vi "Task Manager.vi"(8 "error in (no error)":errorcluster, 11 "Task":string) -> (0 "error out":errorcluster, 3 "Task Properties":T1)   [LabVIEW 2018, in "Main.lvlib"]
uses:
  Main.lvlib
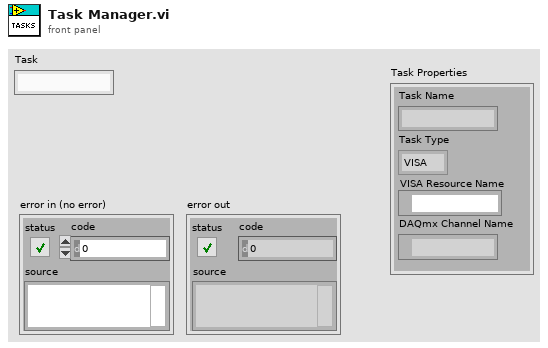
[diagram p1: front panel]
types:
  T1 = cluster{"Task Name":string, "Task Type":enum16{"VISA", "DAQmx"}, "VISA Resource Name":refnum<visa-resource-name>, "DAQmx Channel Name":tag}
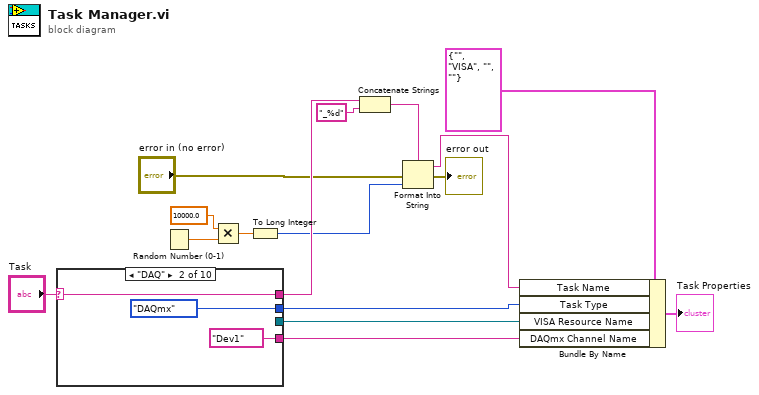
[diagram p0: block diagram]
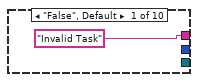
[diagram p2: hidden frame]
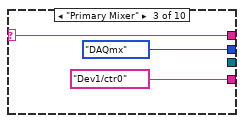
[diagram p3: hidden frame]
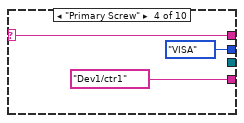
[diagram p4: hidden frame]
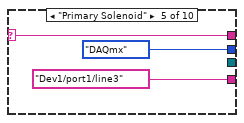
[diagram p5: hidden frame]
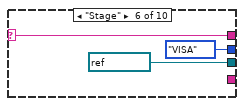
[diagram p6: hidden frame]
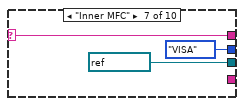
[diagram p7: hidden frame]
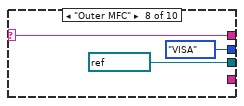
[diagram p8: hidden frame]
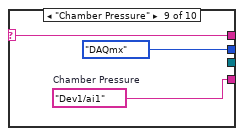
[diagram p9: hidden frame]
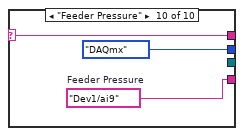
[diagram p10: hidden frame]
diagram:
  n1 = case shown="\"DAQ\"" "Task" {
    selector: "Task" -> [_ w20 w23 w26 w29 w32 w35 w38 w41 w44]
    tunnel: ["Invalid Task" w20 w23 w26 w29 w32 w35 w38 w41 w44] -> w15
    tunnel: [_ _ _ _ _ refnum<visa-resource-name> "COM8" ("VISA resource name") refnum<visa-resource-name> "COM2" ("VISA resource name") refnum<visa-resource-name> "COM1" ("VISA resource name") _ _] -> w4
    tunnel: [_ enum16{"VISA", "DAQmx"}."DAQmx" ("Task Type") enum16{"VISA", "DAQmx"}."DAQmx" ("Task Type") enum16{"VISA", "DAQmx"}."VISA" ("Task Type") enum16{"VISA", "DAQmx"}."DAQmx" ("Task Type") enum16{"VISA", "DAQmx"}."VISA" ("Task Type") enum16{"VISA", "DAQmx"}."VISA" ("Task Type") enum16{"VISA", "DAQmx"}."VISA" ("Task Type") enum16{"VISA", "DAQmx"}."DAQmx" ("Task Type") enum16{"VISA", "DAQmx"}."DAQmx" ("Task Type")] -> w3
    tunnel: [_ tag "Dev1" ("Counter(s)") tag "Dev1/ctr0" ("Counter(s)") tag "Dev1/ctr1" ("Counter(s)") tag "Dev1/port1/line3" ("lines") _ _ _ w40 w43] -> w2
    frame "False", Default {
    }
    frame "DAQ" {
    }
    frame "Primary Mixer" {
    }
    frame "Primary Screw" {
    }
    frame "Primary Solenoid" {
    }
    frame "Stage" {
    }
    frame "Inner MFC" {
    }
    frame "Outer MFC" {
    }
    frame "Chamber Pressure" {
      w40 = tag "Dev1/ai1"  # Chamber Pressure
    }
    frame "Feeder Pressure" {
      w43 = tag "Dev1/ai9"  # Feeder Pressure
    }
  }
  n2 = Random Number (0-1)() -> (number: 0 to 1=w14:dbl)
  n3 = Multiply(x=10000.0, y=w14) -> (x*y=w12:dbl)
  n4 = To Long Integer(number=w12) -> (32bit integer=w11:i32)
  n5 = Concatenate Strings(w15, "_%d" ("string")) -> (w7:string)
  n6 = Format Into String(format string=w7, error in="error in (no error)", w11) -> (resulting string=w5:string, error out=→"error out":errorcluster)  [unwired: 1 in]
  n7 = Bundle By Name(cluster=T1 {"Task Name"="", "Task Type"=enum."VISA", "VISA Resource Name"="", "DAQmx Channel Name"=""} ("Task Output 2"), "Task Name"=w5, "Task Type"=w3, "VISA Resource Name"=w4, "DAQmx Channel Name"=w2) -> (→"Task Properties":T1)
